vi "Keyence LJ-V7000 Read Profiles(for High-Speed Mode).vi"() -> ()   [LabVIEW 2014]
doc: "This example mainly indicates how to acquire profiles from controllers by using <B>Read Profiles (for High-Speed Mode)</B> VI.\n\n<B>Note</B>:\nIf you execute this example, set the operation mode of the controller to the high-speed mode."
uses:
  Public/constant/Comm Interface.ctl
  Public/Clusters/Ethernet Config.ctl
  Public/Clusters/Read Profile Req.ctl
  Public/constant/Profile Pos.ctl
  Public/Clusters/Profile Info.ctl
  Public/Clusters/Read Profile Rsp.ctl
  Keyence LJ-V7000.lvlib
panel:
  out "Profile Monitor":cluster{dbl, dbl, dbl[]}(graph)
  out "Profile Rsp":T1
  out "Profile Info":T2={"Profile Cnt"=1, "Envelope"=FALSE, " Profile Data Point"=0, " X Start"=0, " X Pitch"=0}
  in  "Read Req":T3={"Read Area"=TRUE, "Profile Pos"=0, "Read Profile No."=0, "Read Profile Cnt"=1, "Erase"=FALSE} {"Profile Pos" items=["CURRENT", "OLDEST", "SPECIFY"]}
  in  "Stop VI":bool
  in  "Ethernet Config":T5={"IP Address"=[192, 168, 0, 1], "Port No"=24691}
  in  "Comm Interface":T6
  # "Communication Configuration"
  # "Output from Read Profiles VI"
  # "Input to Read Profiles VI"
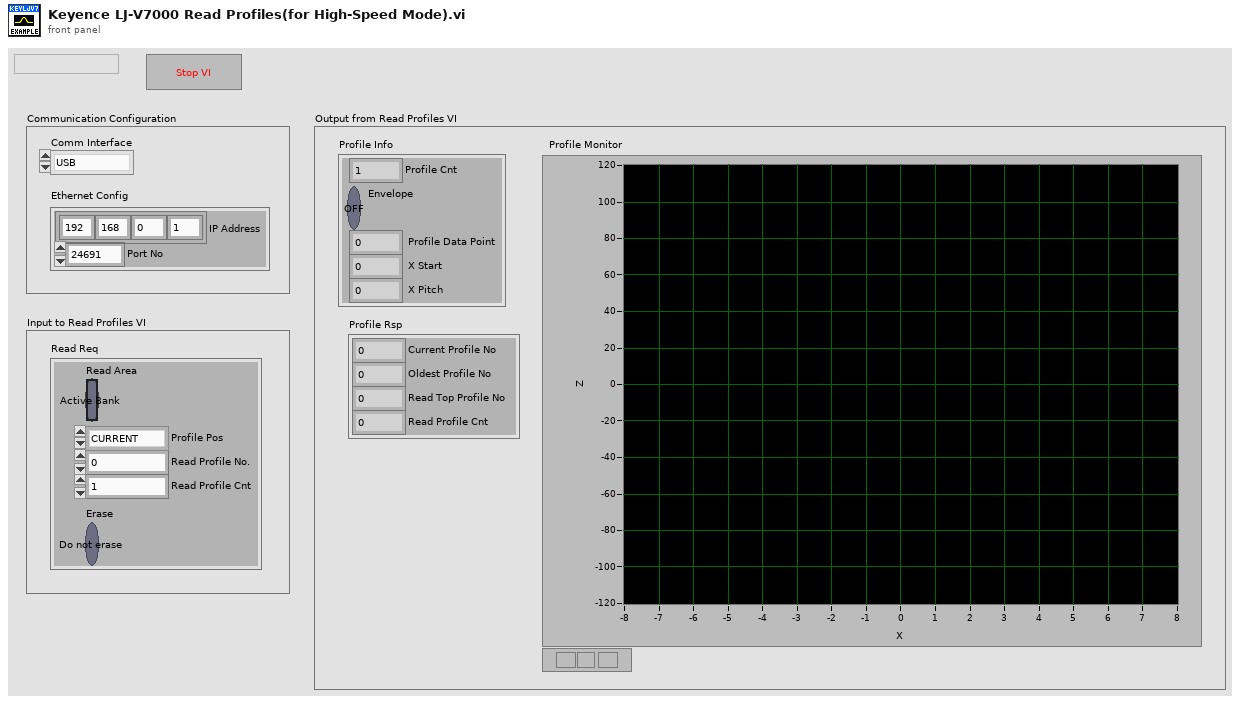
[diagram p1: front panel]
types:
  T1 = typedef "Keyence LJ-V7000.lvlib/Read Profile Rsp.ctl" = cluster{"Current Profile No":u32, "Oldest Profile No":u32, "Read Top Profile No":u32, "Read Profile Cnt":u8}
  T2 = typedef "Keyence LJ-V7000.lvlib/Profile Info.ctl" = cluster{"Profile Cnt":u8, "Envelope":bool, " Profile Data Point":u16, " X Start":i32, " X Pitch":i32}
  T3 = typedef "Keyence LJ-V7000.lvlib/Read Profile Req.ctl" = cluster{"Read Area":bool, "Profile Pos":T4, "Read Profile No.":u32, "Read Profile Cnt":u8, "Erase":bool}
  T4 = typedef "Keyence LJ-V7000.lvlib/Profile Pos.ctl" = u8
  T5 = typedef "Keyence LJ-V7000.lvlib/Ethernet Config.ctl" = cluster{"IP Address":u8[], "Port No":u16}
  T6 = typedef "Keyence LJ-V7000.lvlib/Comm Interface.ctl" = enum8{"USB", "ETHERNET"}
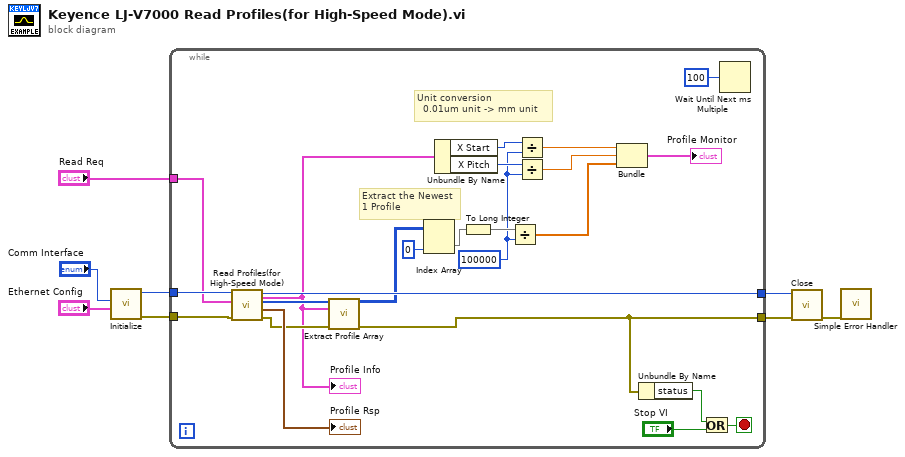
[diagram p0: block diagram]
diagram:
  n1 = call "Initialize.vi"("Ethernet Config"="Ethernet Config", "Comm Interface"="Comm Interface") -> ("error out"=w8:errorcluster, "Device ID out"=w7:i32)  [unwired: 8 in]
  n2 = while {
    tunnel: w8 -> [w30]
    tunnel: w7 -> [w31]
    tunnel: [w9] -> w6
    tunnel: [w28] -> w5
    tunnel: "Read Req" -> [w29]
    stop <- w12 stop-if-true
    w14 = 100000
    # "Extract the Newest\n1 Profile"
    # "Unit conversion\n  0.01um unit -> mm unit"
    n3 = call "Read Profiles(for High-Speed Mode).vi"("error in (no error)"=w30, "Read Req"=w29, "Device ID (0)"=w31) -> ("error out"=w25:errorcluster, "Profile Rsp"=→"Profile Rsp":T1, "Profile Data"=w26:u32[], "Device ID out"=w28:i32, "Profile Info"=w24:T2)  [unwired: 4 in]
    "Profile Info" <- w24
    n4 = call "Extract Profile Array.vi"("Profile Data"=w26, "Profile Info"=w24, "error in (no error)"=w25) -> ("Profile A Array1"=w17:u32[][], "error out"=w9:errorcluster)  [unwired: 8 in, 3 out]
    n5 = Index Array(array=w17, index (col)=0 ("無効な指標 （列）")) -> (element=w16:u32[])  [unwired: 1 in]
    n6 = Unbundle By Name(w24) -> ("X Start"=w23:i32, "X Pitch"=w22:i32)
    n7 = To Long Integer(number=w16) -> (32bit integer=w15:i32[])
    n8 = Divide(x=w15, y=w14) -> (x/y=w13:dbl[])
    n9 = Divide(x=w23, y=w14) -> (x/y=w21:dbl)
    n10 = Divide(x=w22, y=w14) -> (x/y=w20:dbl)
    n11 = Bundle(w21, w20, w13) -> (→"Profile Monitor":cluster{dbl, dbl, dbl[]})  [unwired: 1 in]
    n12 = Unbundle By Name(w9) -> ("status"=w10:bool)
    n13 = Or(x=w10, y="Stop VI") -> (x .or. y?=w12:bool)
    n14 = Wait Until Next ms Multiple(millisecond multiple=u32 100 ("ミリ秒倍数")) -> ()  [unwired: 1 out]
  }
  n15 = call "Close.vi"("error in (no error)"=w6, "Device ID (0)"=w5) -> ("error out"=w1:errorcluster)  [unwired: 8 in, 1 out]
  n16 = call <vilib>:"Simple Error Handler.vi"("error in (no error)"=w1) -> ()  [unwired: 4 in, 5 out]
